vi "Image Example.vi"() -> ()   [LabVIEW 2012]
uses:
  Non-User VIs/Controls/Image Parameters.ctl
  Non-User VIs/Images/Channel Order.ctl
  User Controls/Array Dimensions.ctl
  Non-User VIs/Images/Data Type.ctl
  User Controls/Offset.ctl
  OpenCLV x64.lvlib
panel:
  in  "Image Parameters":T1={"Channel Order"=enum."CL_LUMINANCE (Grayscale)", "Dimension"={"Depth"=1, "Height"=1024, "Width"=1024}, "Data Type"=enum."32f", "Offset"={"X"=0, "Y"=0, "Z"=0}} {"Dimension"."Width" min=1; "Dimension"."Height" min=1; "Dimension"."Depth" min=1}
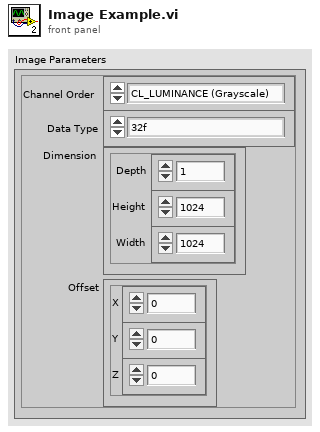
[diagram p1: front panel]
types:
  T1 = typedef "OpenCLV x64.lvlib/Image Parameters.ctl" = cluster{"Channel Order":T2, "Dimension":T3, "Data Type":T4, "Offset":T5}
  T2 = typedef "OpenCLV x64.lvlib/Channel Order.ctl" = enum16{"CL_LUMINANCE (Grayscale)", "CL_INTENSITY (Opacity)", "CL_RGBA", "CL_ARGB", "CL_BGRA", "CL_RG", "CL_RA", "CL_R", "CL_A"}
  T3 = typedef "Array Dimensions.ctl" = cluster{"Depth":u64, "Height":u64, "Width":u64}
  T4 = typedef "OpenCLV x64.lvlib/Data Type.ctl" = enum16{"32f", "u8", "u16", "u32", "i8", "i16", "i32"}
  T5 = typedef "Offset.ctl" = cluster{"X":u64, "Y":u64, "Z":u64}
  T6 = typedef "OpenCLV x64.lvlib/Device ID.ctl" = u64
  T7 = typedef "OpenCLV x64.lvlib/Image Object.ctl" = cluster{"Device ID":T6, "Memeroy ID":T8, "Image Parameters":T1}
  T8 = typedef "OpenCLV x64.lvlib/Memory ID.ctl" = u64
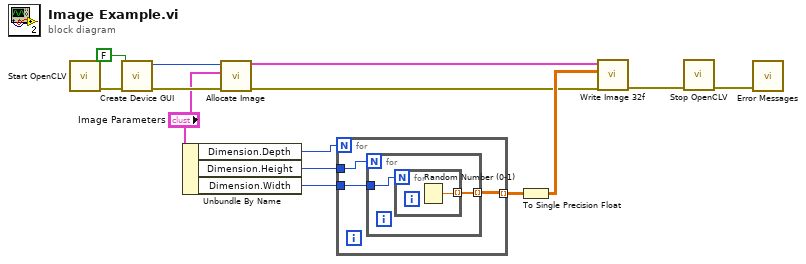
[diagram p0: block diagram]
diagram:
  n1 = call "Start OpenCLV.vi"() -> ("Error Out"=w14:errorcluster)  [unwired: 11 in]
  n2 = call "Create Device GUI.vi"("Error In"=w14, "Skip Configuration"=FALSE) -> ("error constant"=w12:errorcluster, "Device Reference"=w11:T6)  [unwired: 8 in]
  n3 = Unbundle By Name("Image Parameters") -> ("Dimension.Depth"=w9:u64, "Dimension.Height"=w8:u64, "Dimension.Width"=w7:u64)
  n4 = call "Allocate Image.vi"("Error In"=w12, "Image Parameters"="Image Parameters", "Labview Device"=w11) -> ("Error Out"=w1:errorcluster, "Image Object"=w4:T7)  [unwired: 6 in, 1 out]
  n5 = for {
    N: w9 -> [_]
    tunnel: w8 -> [w17]
    tunnel: w7 -> [w16]
    tunnel: [w15] -> w6 mode=indexing
    n6 = for {
      N: w17 -> [_]
      tunnel: w16 -> [w19]
      tunnel: [w18] -> w15 mode=indexing
      n7 = for {
        N: w19 -> [_]
        tunnel: [w20] -> w18 mode=indexing
        n8 = Random Number (0-1)() -> (number: 0 to 1=w20:dbl)
      }
    }
  }
  n9 = To Single Precision Float(number=w6) -> (single precision float=w5:sgl[][][])
  n10 = call "Write Image 32f.vi"("Error In"=w1, "Data"=w5, "Image Object"=w4) -> ("Error Out"=w3:errorcluster)  [unwired: 6 in, 2 out]
  n11 = call "Stop OpenCLV.vi"("Error In"=w3) -> ("Error Out"=w2:errorcluster)  [unwired: 10 in]
  n12 = call "Error Messages.vi"("error in (no error)"=w2) -> ()  [unwired: 9 in, 2 out]
